vi "XML ( Get Node Value Multiple Inputs ).vi"(8 "error in (no error)":errorcluster, 10 "XPath expression":string[](array[string]), 11 "XML in":refnum<class "XML.lvclass">) -> (0 "error out":errorcluster, 2 "Value":string[](array[string]), 3 "XML out":refnum<class "XML.lvclass">)   [LabVIEW 2018, in "XML.lvlib" / "XML.lvclass"]
uses:
  XML.lvclass
  XML.lvclass/XML.ctl
  <vilib>/xml/Close Reference(Node).vi
  <vilib>/xml/NI_XML.lvlib
  <resource>/objmgr/DOMUserDefRef.rc
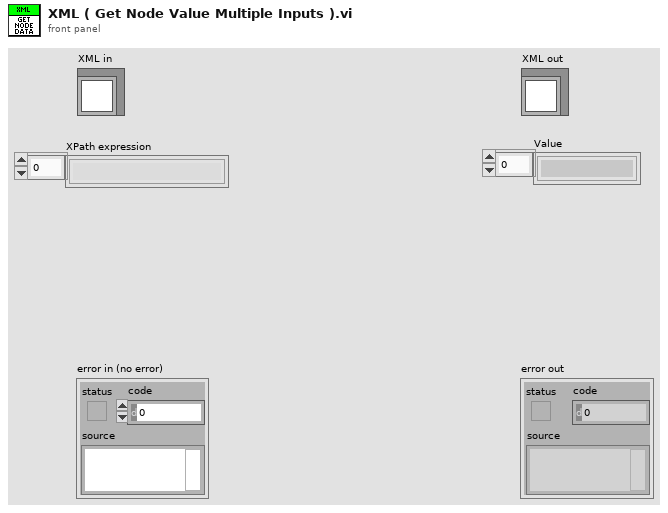
[diagram p1: front panel]
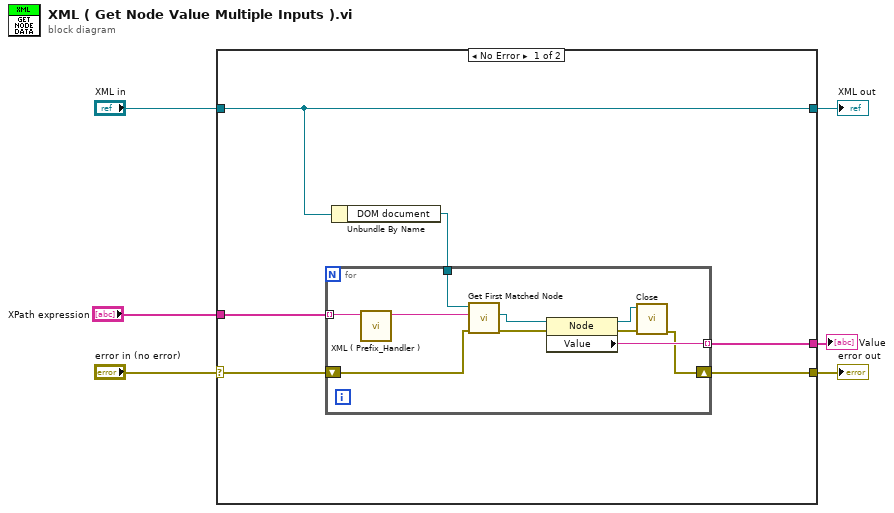
[diagram p0: block diagram]
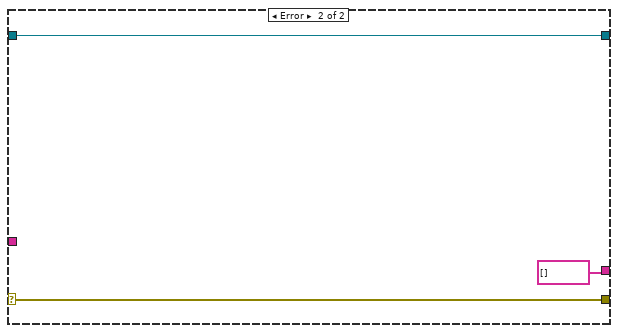
[diagram p2: hidden frame]
diagram:
  n1 = case shown="No Error" "error in (no error)" {
    selector: "error in (no error)" -> [w10 w25]
    tunnel: [w8 w25] -> w5
    tunnel: [w12 w24] -> w3
    tunnel: "XML in" -> [w12 w24]
    tunnel: [w9 string[] []] -> w2
    tunnel: "XPath expression" -> [w7 _]
    frame No Error {
      n2 = Unbundle By Name(w12) -> ("DOM document"=w11:refnum<k20>)
      n3 = for {
        tunnel: w11 -> [w20]
        tunnel: [w16] -> w9 mode=indexing
        tunnel: w7 -> [w14] mode=indexing
        shift-right: [w15] -> w8
        shift-left: w10 -> [w19]
        n4 = call "XML ( Prefix_Handler ).vi"("input string"=w14) -> ("result string"=w13:string)  [unwired: 10 in]
        n5 = call <vilib>:"Get First Matched Node.vi"("error in (no error)"=w19, "XPath expression"=w13, "node in"=w20) -> ("error out"=w21:errorcluster, "node result"=w22:refnum<k20>)  [unwired: 6 in, 1 out]
        n6 = property class="Node"(reference=w22, error in=w21) -> (reference out=w17:refnum<k20>, error out=w18:errorcluster, "Value"=w16:string)
        n7 = call-poly <vilib>:"Close.vi"("error in (no error)"=w18, "node"=w17) -> ("error out"=w15:errorcluster)  [unwired: 7 in]
      }
    }
    frame Error {
    }
  }
  "error out" <- w5
  "XML out" <- w3
  "Value" <- w2
